vi "Value to U8 string.vi"(1 "Value":u8) -> (0 "U8 str":string)   [LabVIEW 2015]
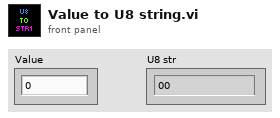
[diagram p1: front panel]
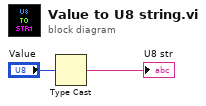
[diagram p0: block diagram]
diagram:
  n1 = Type Cast(x="Value") -> (*(type *) &x=→"U8 str":string)  [unwired: 1 in]
